vi "Monitor Interface Error.vi"(8 "error in":errorcluster, 11 "3300 in":refnum<class "3300.lvclass">) -> (0 "error out":errorcluster, 3 "3300 out":refnum<class "3300.lvclass">)   [LabVIEW 2019, in "3300.lvlib" / "3300.lvclass"]
uses:
  Library/3300.lvclass
  Library/3300.lvclass/3300.ctl
  <instrlib>/Agilent N330X Series/Agilent N330X Series.lvlib
  builds/Engine/Engine.lvlibp/Project/Engine.lvclass
  C:/Users/Public/Documents/Development/builds/Engine/Engine.lvlibp/Project/Engine.lvclass
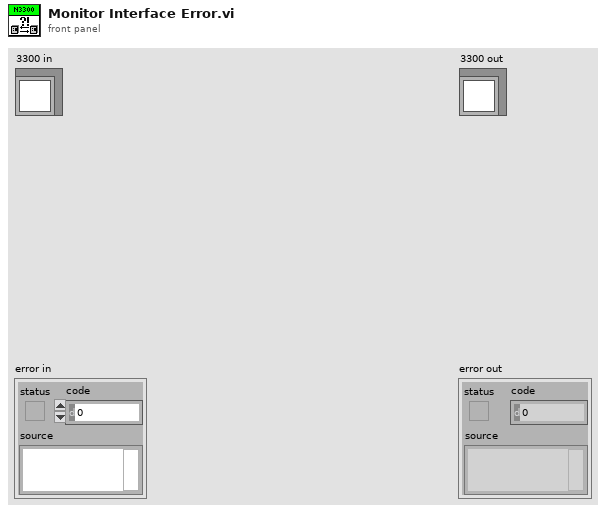
[diagram p1: front panel]
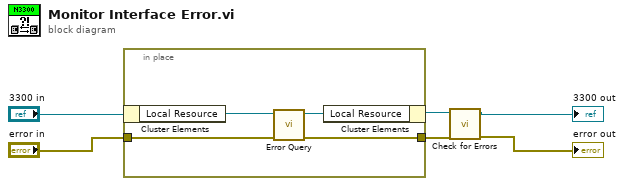
[diagram p0: block diagram]
diagram:
  n1 = in-place {
    in-place-border: "error in" -> [w7]
    in-place-border: [w8] -> w4
    n2 = in-place-cluster #1("3300 in") -> ("Local Resource"=w10:refnum<visa-resource-name>)
    n3 = call <instrlib>:"Error Query.vi"("error in (no error)"=w7, "VISA resource name"=w10) -> ("error out"=w8:errorcluster, "VISA resource name out"=w9:refnum<visa-resource-name>)  [unwired: 6 in, 2 out]
    n4 = in-place-cluster #1("Local Resource"=w9) -> (w3:refnum<class "3300.lvclass">)
  }
  n5 = call "Check for Errors.vi"("error in"=w4, "Engine in"=w3) -> ("error out"=→"error out":errorcluster, "Engine out"=→"3300 out":refnum<class "3300.lvclass">)  [unwired: 8 in]
